vi "Process.vi"(8 "error in (no error)":errorcluster, 10 "Wait for Start State in":refnum<class "Wait for Start State.lvclass">, 11 "Architecture.lvlib:Thread.lvclass":refnum<class "Thread.lvclass">) -> (0 "error out":errorcluster, 1 "Stop?":bool, 3 "Architecture.lvlib:Thread.lvclass 2":refnum<class "Thread.lvclass">)   [LabVIEW 2012, in "Car Wash Controller.lvlib" / "Wait for Start State.lvclass"]
uses:
  Wait for Start State.lvclass
  Message/Message.lvclass
  Thread/Thread.lvclass
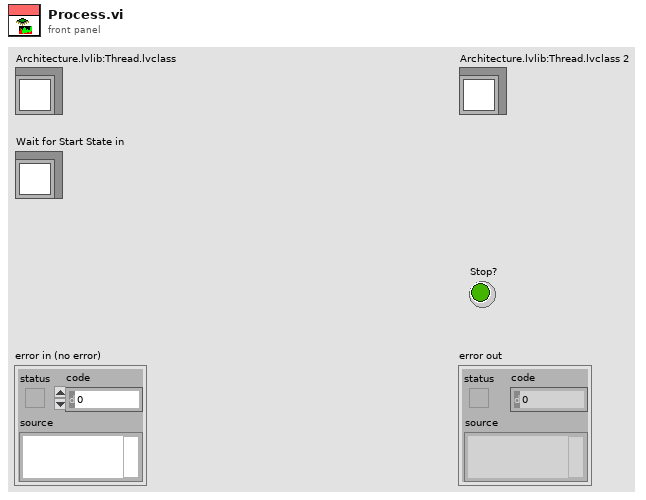
[diagram p1: front panel]
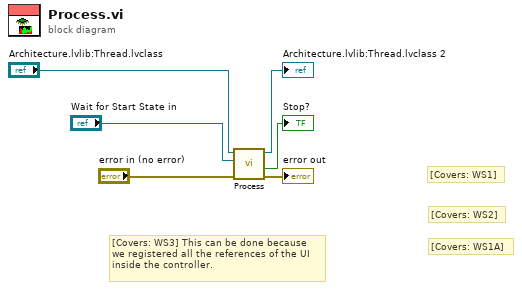
[diagram p0: block diagram]
diagram:
  # "[Covers: WS3] This can be done because\nwe registered all the references of the UI\ninside the controller."
  # "[Covers: WS1A]"
  # "[Covers: WS2]"
  # "[Covers: WS1]"
  n1 = call-parent "Process.vi"("error in (no error)"="error in (no error)", "Message in"="Wait for Start State in", "Architecture.lvlib:Thread.lvclass"="Architecture.lvlib:Thread.lvclass") -> ("error out"=→"error out":errorcluster, "Stop?"=→"Stop?":bool, "Architecture.lvlib:Thread.lvclass 2"=→"Architecture.lvlib:Thread.lvclass 2":refnum<class "Thread.lvclass">)  [unwired: 6 in]
